vi "HDLC Synchronous Acquire.vi"(2 "Clock":bool[](array[boolean]), 3 "Min PW of Clock in samples":i32=60, 4 "Data":bool[](array[boolean]), 5 "Invert data(T)":bool) -> (1 "Data Out":bool[](array[boolean]))   [LabVIEW 2019]
doc: "HDLC is a bit - oriented protocol where each frame contains up to six fields. \nThis VI samples data on the basis of clock.\nCurrently it is Configured for Detection at mid point of Clock Pulse Width.\nIt can be configured at Rising or Falling Edge of Clock. \nRefer to Comments on the block diagram of this VI."
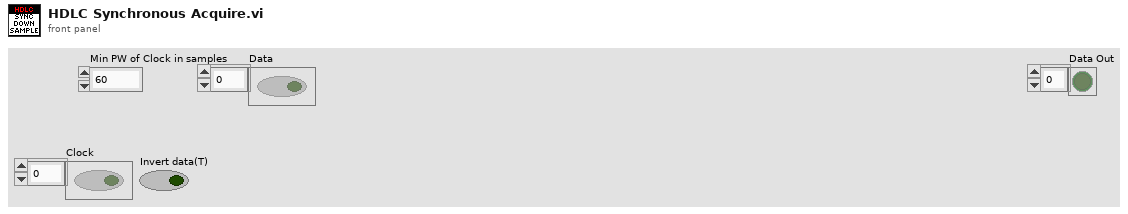
[diagram p1: front panel]
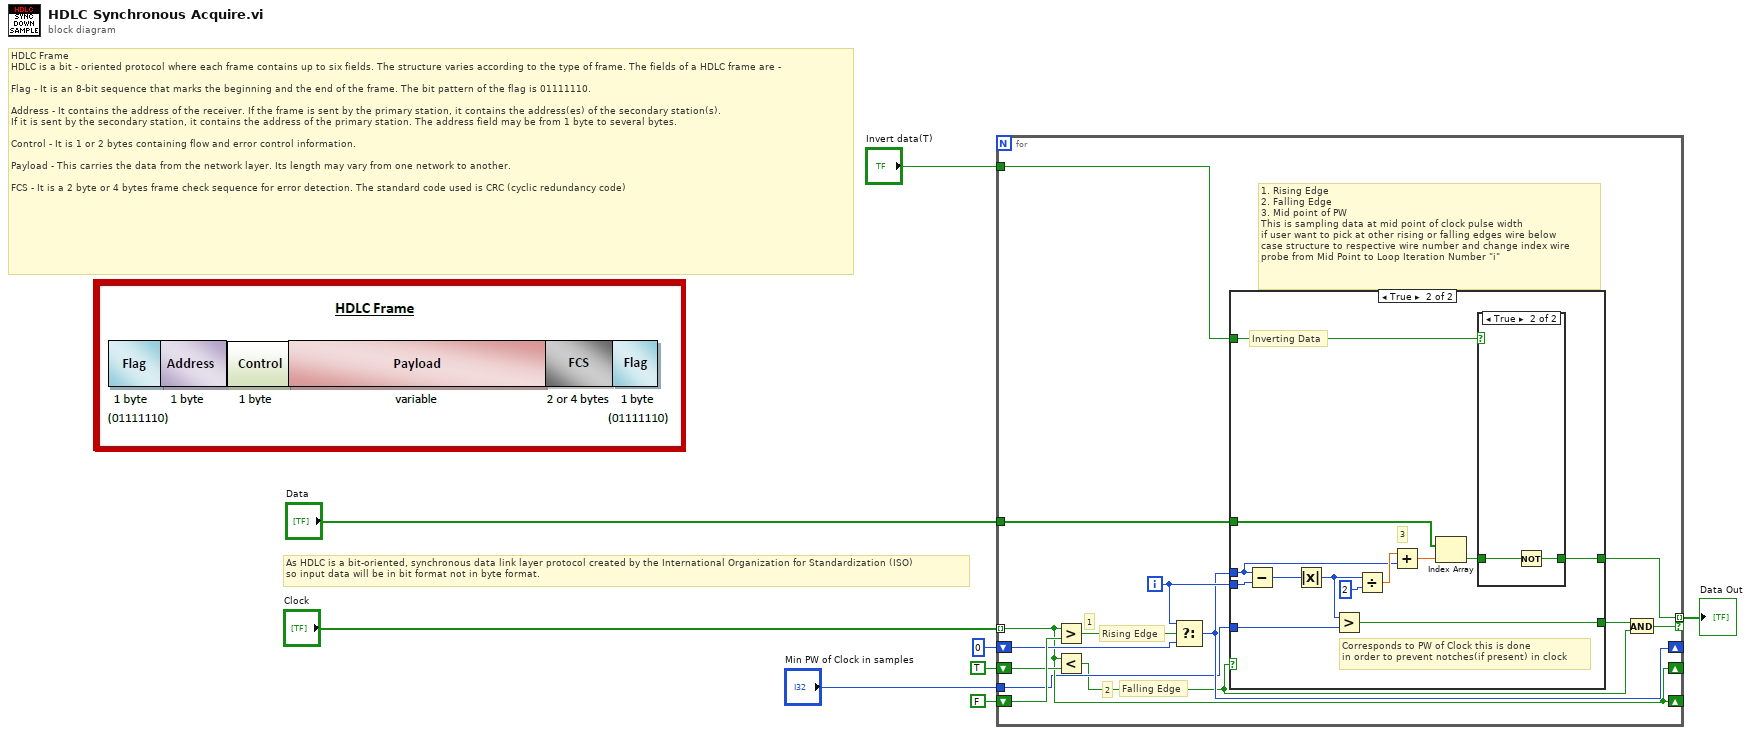
[diagram p0: block diagram]
diagram:
  # "HDLC Frame\nHDLC is a bit - oriented protocol where each frame contains up to six fields. The structure varies according to the type of frame. The fields of a HDLC frame are -\n\nFlag - It is an 8-bit sequence that marks the beginning and the end of the frame. The bit pattern of the flag is 01111110.\n\nAddress - It contains the address of the receiver. If the frame is sent by the primary station, it contains the address(es) of the secondary station(s). \nIf it is sent by the secondary station, it contains the address of the primary station. The address field may be from 1 byte to several bytes.\n\nControl - It is 1 or 2 bytes containing flow and error control information.\n\nPayload - This carries the data from the network layer. Its length may vary from one network to another.\n\nFCS - It is a 2 byte or 4 bytes frame check sequence for error detection. The standard code used is CRC (cyclic redundancy code)"
  # "As HDLC is a bit-oriented, synchronous data link layer protocol created by the International Organization for Standardization (ISO)\nso input data will be in bit format not in byte format."
  n1 = for {
    tunnel: "Clock" -> [w12] mode=indexing
    shift-right: [w12] -> _
    shift-left: FALSE -> [w22]
    tunnel: "Data" -> [w20]
    tunnel: [w19] -> w6 mode=indexing if=w18
    shift-right: [w12] -> _
    shift-left: TRUE -> [w21]
    shift-right: [w13] -> _
    shift-left: 0 -> [w14]
    tunnel: "Min PW of Clock in samples" -> [w11]
    tunnel: "Invert data(T)" -> [w10]
    i -> [w15]
    # "Falling Edge"
    # "Rising Edge"
    # "2"
    # "1"
    # "1. Rising Edge\n2. Falling Edge\n3. Mid point of PW\nThis is sampling data at mid point of clock pulse width \nif user want to pick at other rising or falling edges wire below \ncase structure to respective wire number and change index wire \nprobe from Mid Point to Loop Iteration Number \"i\""
    n2 = Greater?(x=w12, y=w22) -> (0:w16:bool)
    n3 = Less?(x=w12, y=w21) -> (x < y?=w9:bool)
    n4 = Select(t=w15, s=w16, f=w14) -> (s? t:f=w13:i32)
    n5 = case shown="True" w9 {
      tunnel: w15 -> [_ w32]
      tunnel: [_ w35] -> w19
      tunnel: w20 -> [_ w33]
      tunnel: [_ w25] -> w17
      tunnel: w13 -> [_ w26]
      tunnel: w11 -> [_ w24]
      tunnel: w10 -> [_ w23]
      frame False {
      }
      frame True {
        # "3"
        # "Inverting Data"
        # "Corresponds to PW of Clock this is done\nin order to prevent notches(if present) in clock"
        n6 = Subtract(x=w26, y=w32) -> (x-y=w34:i32)
        n7 = Absolute Value(x=w34) -> (abs(x)=w27:i32)
        n8 = Greater?(x=w27, y=w24) -> (0:w25:bool)
        n9 = Divide(x=w27, y=2 ("x")) -> (x/y=w30:dbl)
        n10 = Add(x=w30, y=w26) -> (x+y=w28:dbl)
        n11 = Index Array(array=w33, index=w28) -> (element=w31:bool)
        n12 = case shown="True" w23 {
          tunnel: [w36 w37] -> w35
          tunnel: w31 -> [w36 w38]
          frame False {
          }
          frame True {
            n13 = Not(x=w38) -> (.not. x?=w37:bool)
          }
        }
      }
    }
    n14 = And(x=w17, y=w9) -> (x .and. y?=w18:bool)
  }
  "Data Out" <- w6
